vi "ChaseBoat.vi"(3 "Base Station data rec'd":string, 4 "inPriors":T1(array[cluster]), 5 "Tug letter":string="G") -> (0 "outPriors":T1(array[cluster]), 1 "predictedY":dbl, 2 "predictedX":dbl)   [LabVIEW 2012]
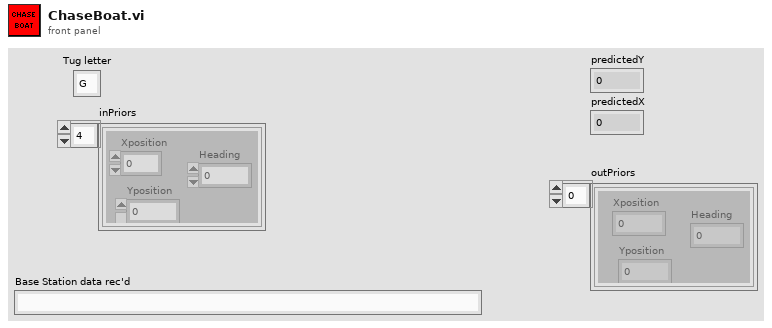
[diagram p1: front panel]
types:
  T1 = cluster{"Xposition":dbl, "Yposition":dbl, "Heading":dbl}[]
  T2 = cluster{"regular expression":string, i32, i32, i32}
  T3 = cluster{"Xposition":dbl, "Yposition":dbl, "Heading":dbl}
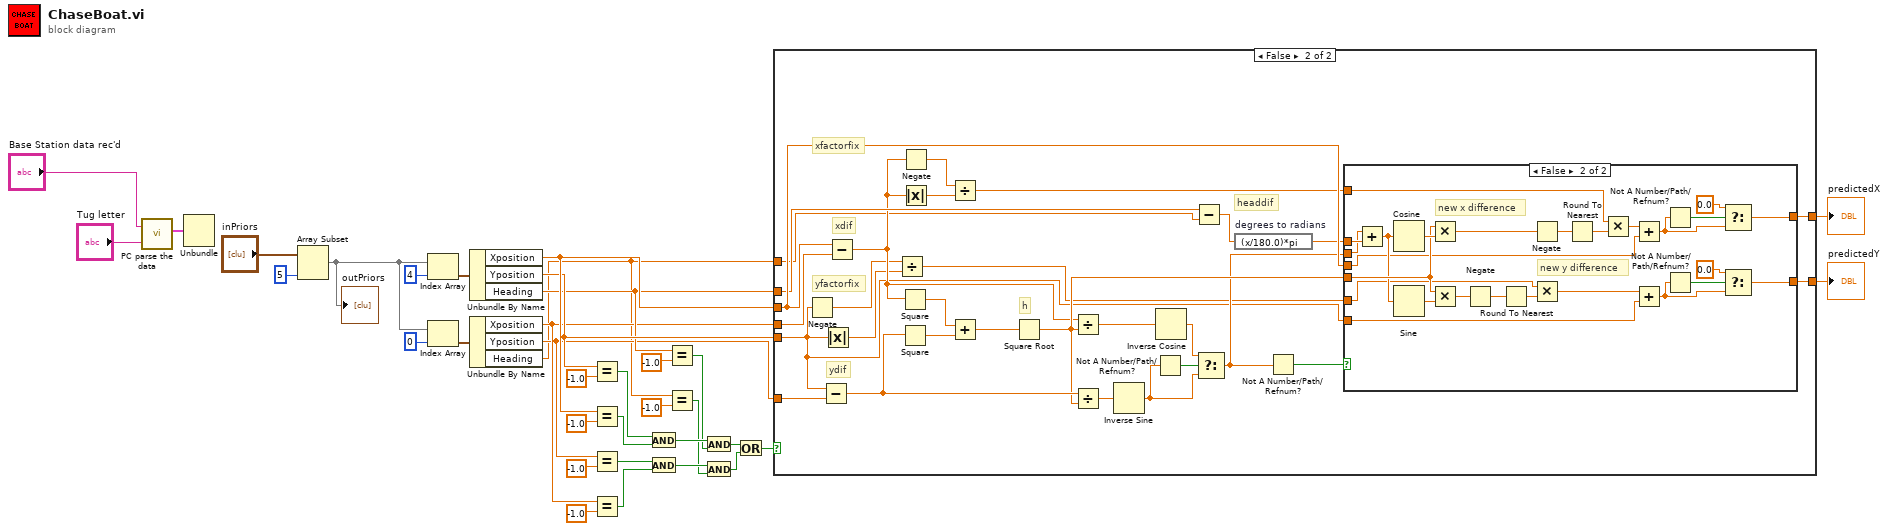
[diagram p0: block diagram]
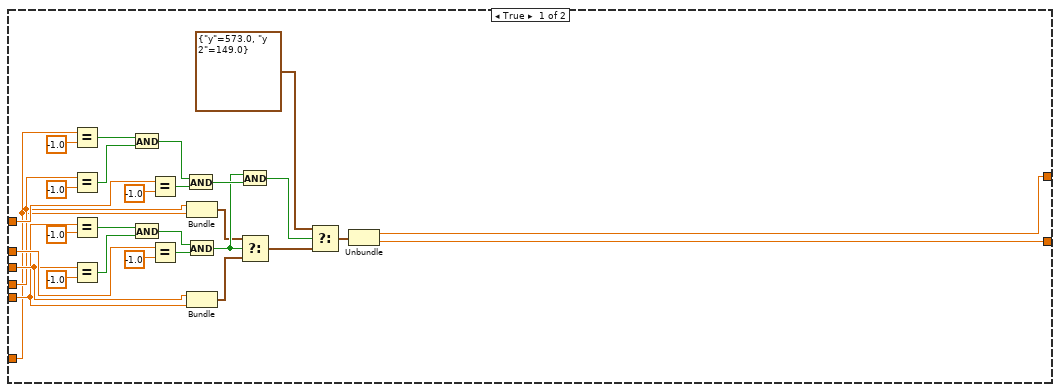
[diagram p2: hidden frame]
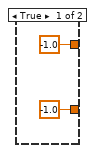
[diagram p3: hidden frame]
diagram:
  n1 = call "PC parse the data.vi"("Nav String"="Base Station data rec'd", "Tug"="Tug letter") -> ("Tug Location"=w33:T2)  [unwired: 3 out]
  n2 = Unbundle(w33) -> ()  [unwired: 4 out]
  n3 = Array Subset(array="inPriors", length=5) -> (w31:T1)  [unwired: 1 in]
  "outPriors" <- w31
  n4 = Index Array(array=w31, index=4) -> (element=w27:T3)
  n5 = Index Array(array=w31, index=0) -> (element=w28:T3)
  n6 = Unbundle By Name(w27) -> ("Xposition"=w6:dbl, "Yposition"=w5:dbl, "Heading"=w4:dbl)
  n7 = Unbundle By Name(w28) -> ("Xposition"=w3:dbl, "Yposition"=w2:dbl, "Heading"=w1:dbl)
  n8 = Equal?(x=w5, y=-1.0) -> (x = y?=w22:bool)
  n9 = Equal?(x=w6, y=-1.0) -> (x = y?=w23:bool)
  n10 = Equal?(x=w2, y=-1.0) -> (x = y?=w15:bool)
  n11 = Equal?(x=w3, y=-1.0) -> (x = y?=w16:bool)
  n12 = And(x=w22, y=w23) -> (x .and. y?=w21:bool)
  n13 = And(x=w15, y=w16) -> (x .and. y?=w14:bool)
  n14 = Equal?(x=w4, y=-1.0) -> (x = y?=w20:bool)
  n15 = Equal?(x=w1, y=-1.0) -> (x = y?=w13:bool)
  n16 = And(x=w21, y=w20) -> (x .and. y?=w8:bool)
  n17 = And(x=w14, y=w13) -> (x .and. y?=w9:bool)
  n18 = Or(x=w8, y=w9) -> (x .or. y?=w7:bool)
  n19 = case shown="False" w7 {
    tunnel: w3 -> [w42 w94]
    tunnel: w2 -> [w41 w93]
    tunnel: w6 -> [w45 w89]
    tunnel: [w36 w88] -> w25
    tunnel: [w37 w87] -> w24
    tunnel: w4 -> [w58 w76]
    tunnel: w5 -> [w44 w69]
    tunnel: w1 -> [w50 w66]
    frame True {
      n20 = Equal?(x=w41, y=-1.0) -> (x = y?=w56:bool)
      n21 = Equal?(x=w42, y=-1.0) -> (x = y?=w57:bool)
      n22 = Equal?(x=w44, y=-1.0) -> (x = y?=w64:bool)
      n23 = Equal?(x=w45, y=-1.0) -> (x = y?=w65:bool)
      n24 = And(x=w56, y=w57) -> (x .and. y?=w55:bool)
      n25 = And(x=w64, y=w65) -> (x .and. y?=w63:bool)
      n26 = Equal?(x=w50, y=-1.0) -> (x = y?=w54:bool)
      n27 = Equal?(x=w58, y=-1.0) -> (x = y?=w62:bool)
      n28 = And(x=w55, y=w54) -> (x .and. y?=w49:bool)
      n29 = Bundle("Xposition"=w42, "Yposition"=w41) -> (w40:cluster{"Xposition":dbl, "Yposition":dbl})  [unwired: 1 in]
      n30 = And(x=w63, y=w62) -> (x .and. y?=w46:bool)
      n31 = Bundle("Xposition"=w45, "Yposition"=w44) -> (w43:cluster{"Xposition":dbl, "Yposition":dbl})  [unwired: 1 in]
      n32 = And(x=w46, y=w49) -> (x .and. y?=w48:bool)
      n33 = Select(t=w40, s=w46, f=w43) -> (s? t:f=w39:cluster{"Xposition":dbl, "Yposition":dbl})
      n34 = Select(t=cluster{"y":dbl, "y 2":dbl} {"y"=573.0, "y 2"=149.0}, s=w48, f=w39) -> (s? t:f=w38:cluster{"Xposition":dbl, "Yposition":dbl})
      n35 = Unbundle(w38) -> ("Xposition"=w37:dbl, "Yposition"=w36:dbl)
    }
    frame False {
      # "yfactorfix"
      # "xfactorfix"
      # "h"
      # "xdif"
      # "ydif"
      # "headdif"
      n36 = Negate(x=w69) -> (-x=w71:dbl)
      n37 = Subtract(x=w69, y=w93) -> (x-y=w85:dbl)
      n38 = Absolute Value(x=w69) -> (abs(x)=w70:dbl)
      n39 = Subtract(x=w89, y=w94) -> (x-y=w74:dbl)
      n40 = Divide(x=w71, y=w70) -> (x/y=w68:dbl)
      n41 = Square(x=w74) -> (x^2=w92:dbl)
      n42 = Square(x=w85) -> (x^2=w91:dbl)
      n43 = Negate(x=w74) -> (-x=w73:dbl)
      n44 = Absolute Value(x=w74) -> (abs(x)=w72:dbl)
      n45 = Divide(x=w73, y=w72) -> (x/y=w67:dbl)
      n46 = Add(x=w92, y=w91) -> (x+y=w90:dbl)
      n47 = Square Root(x=w90) -> (sqrt(x)=w84:dbl)
      n48 = Divide(x=w74, y=w84) -> (x/y=w86:dbl)
      n49 = Divide(x=w85, y=w84) -> (x/y=w83:dbl)
      n50 = Inverse Sine(1:w83) -> (0:w81:dbl)
      n51 = Not A Number/Path/Refnum?(number/path/refnum=w81) -> (NaN/Path/Refnum?=w82:bool)
      n52 = Inverse Cosine(1:w86) -> (0:w80:dbl)
      n53 = Subtract(x=w76, y=w66) -> (x-y=w75:dbl)
      n54 = Select(t=w80, s=w82, f=w81) -> (s? t:f=w77:dbl)
      n55 = expression code="(x/180.0)*pi" "degrees to radians"(w75) -> (w79:dbl)
      n56 = Not A Number/Path/Refnum?(number/path/refnum=w77) -> (NaN/Path/Refnum?=w78:bool)
      n57 = case shown="False" w78 {
        tunnel: w89 -> [_ w113]
        tunnel: [-1.0 w104] -> w88
        tunnel: w69 -> [_ w114]
        tunnel: [-1.0 w101] -> w87
        tunnel: w84 -> [_ w118]
        tunnel: w79 -> [_ w117]
        tunnel: w77 -> [_ w116]
        tunnel: w68 -> [_ w99]
        tunnel: w67 -> [_ w110]
        frame True {
        }
        frame False {
          # "new x difference"
          # "new y difference"
          n58 = Add(x=w116, y=w117) -> (x+y=w115:dbl)
          n59 = Cosine(x=w115) -> (cos(x)=w121:dbl)
          n60 = Sine(x=w115) -> (sin(x)=w122:dbl)
          n61 = Multiply(x=w118, y=w121) -> (x*y=w98:dbl)
          n62 = Multiply(x=w118, y=w122) -> (x*y=w120:dbl)
          n63 = Negate(x=w120) -> (-x=w119:dbl)
          n64 = Round To Nearest(number=w119) -> (nearest integer value=w112:dbl)
          n65 = Negate(x=w98) -> (-x=w97:dbl)
          n66 = Multiply(x=w99, y=w112) -> (x*y=w111:dbl)
          n67 = Round To Nearest(number=w97) -> (nearest integer value=w109:dbl)
          n68 = Multiply(x=w110, y=w109) -> (x*y=w108:dbl)
          n69 = Add(x=w108, y=w113) -> (x+y=w100:dbl)
          n70 = Add(x=w111, y=w114) -> (x+y=w105:dbl)
          n71 = Not A Number/Path/Refnum?(number/path/refnum=w100) -> (NaN/Path/Refnum?=w103:bool)
          n72 = Not A Number/Path/Refnum?(number/path/refnum=w105) -> (NaN/Path/Refnum?=w107:bool)
          n73 = Select(t=0.0, s=w103, f=w100) -> (s? t:f=w101:dbl)
          n74 = Select(t=0.0, s=w107, f=w105) -> (s? t:f=w104:dbl)
        }
      }
    }
  }
  "predictedY" <- w25
  "predictedX" <- w24
